vi "GoTo.vi"(6 "Reinitialize":bool, 10 "Target":dbl[](array[numeric]), 11 "Position":dbl[](array[numeric])) -> (3 "Output\nVelocity":dbl[](array[numeric]) format="%.2f")   [LabVIEW 2016]
uses:
  <vilib>/Analysis/coordinate.llb/2D Cartesian Coordinate Rotation (Scalar).vi
  <vilib>/addons/control/pid/pid.llb/PID (DBL Array).vi
  <vilib>/addons/control/pid/NI_PID_pid.lvlib
  <vilib>/Analysis/NI_AALPro.lvlib
panel:
  out "ERROR W":dbl(graph)
  out "ERROR Y":dbl(graph)
  out "ERROR X":dbl(graph)
  in  "output range":cluster{"output high":dbl, "output low":dbl}[](array[cluster])=[{"output high"=0.88, "output low"=-0.88}, {"output high"=0.88, "output low"=-0.88}, {"output high"=1.0, "output low"=-1.0}]
  in  "PID gains":T1(array[cluster])=[{"proportional gain (Kc)"=0.0012, "integral time (Ti, min)"=0.0, "derivative time (Td, min)"=0.0}, {"proportional gain (Kc)"=1.5, "integral time (Ti, min)"=0.0, "derivative time (Td, min)"=0.0}]
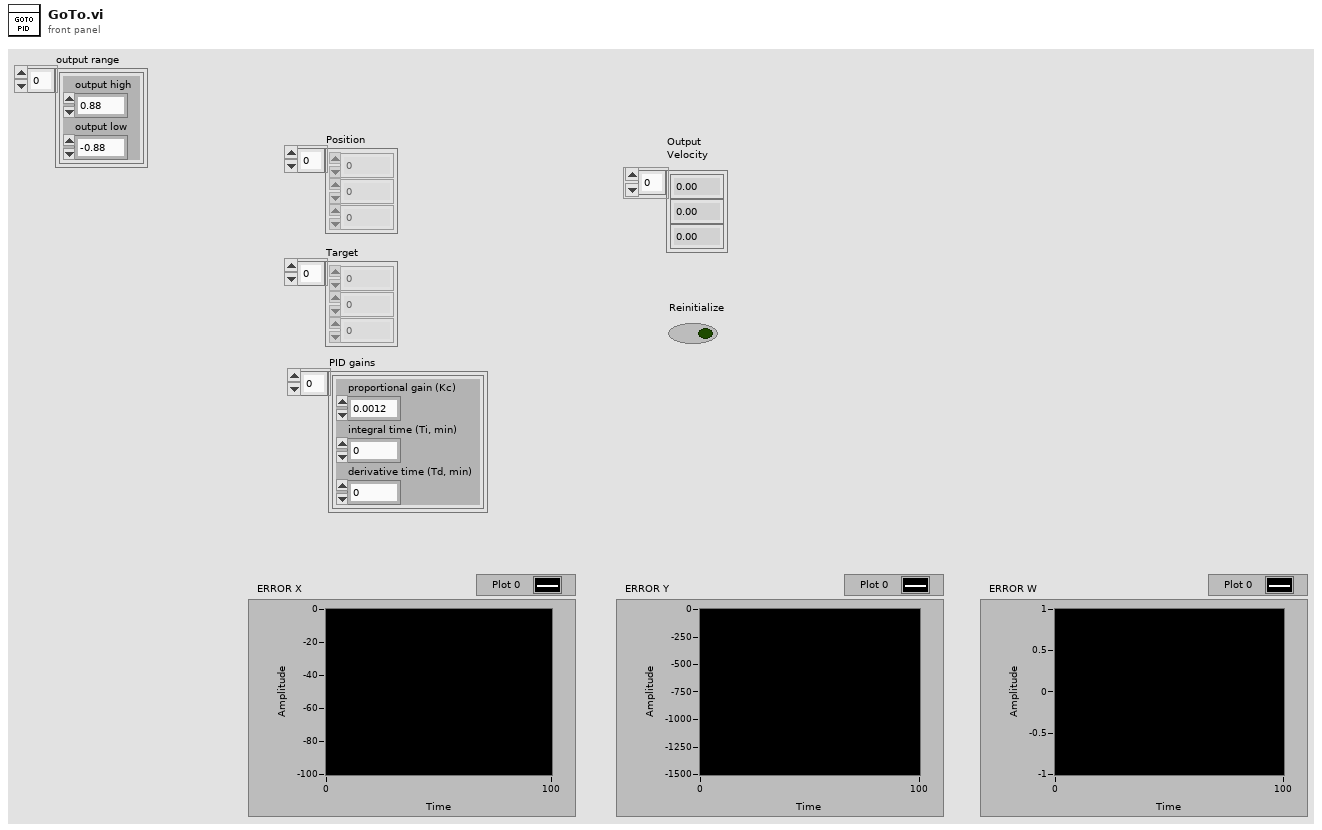
[diagram p1: front panel]
types:
  T1 = cluster{"proportional gain (Kc)":dbl, "integral time (Ti, min)":dbl, "derivative time (Td, min)":dbl}[]
  T2 = cluster{"proportional gain (Kc)":dbl, "integral time (Ti, min)":dbl, "derivative time (Td, min)":dbl}
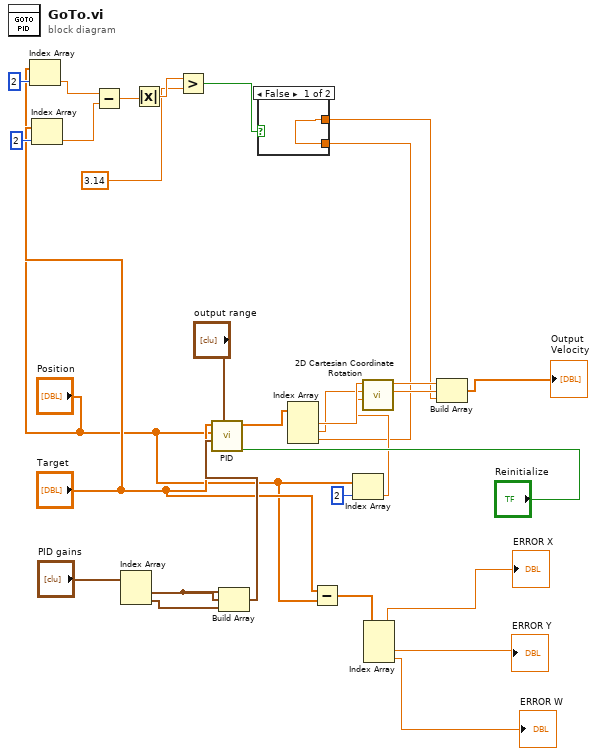
[diagram p0: block diagram]
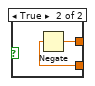
[diagram p2: hidden frame]
diagram:
  n1 = Index Array(array="Position", index=2) -> (element=w14:dbl)
  n2 = Index Array(array="Target", index=2) -> (element=w13:dbl)
  n3 = Subtract(x=w14, y=w13) -> (x-y=w12:dbl)
  n4 = Index Array(array="PID gains") -> (element #1=w19:T2, element #2=w18:T2)  [unwired: 2 in]
  n5 = Absolute Value(x=w12) -> (abs(x)=w11:dbl)
  n6 = Greater?(x=w11, y=3.14) -> (0:w9:bool)
  n7 = Build Array(w19, w19, w18) -> (w17:T1)
  n8 = call-poly <vilib>:"PID.vi"("reinitialize? (F)"="Reinitialize", "output range"="output range", "PID gains"=w17, "process variable"="Position", "setpoint"="Target") -> ("output"=w28:dbl[])  [unwired: 5 in, 1 out]
  n9 = Index Array(array=w28) -> (element #1=w27:dbl, element #2=w26:dbl, element #3=w8:dbl)  [unwired: 3 in]
  n10 = case shown="False" w9 {
    tunnel: w8 -> [w31 w33]
    tunnel: [w31 w32] -> w7
    frame False {
    }
    frame True {
      n11 = Negate(x=w33) -> (-x=w32:dbl)
    }
  }
  n12 = Subtract(x="Target", y="Position") -> (x-y=w4:dbl[])
  n13 = Index Array(array="Position", index=2) -> (element=w21:dbl)
  n14 = call-poly <vilib>:"2D Cartesian Coordinate Rotation.vi"("theta"=w21, "y"=w26, "x"=w27) -> ("y out"=w24:dbl, "x out"=w25:dbl)  [unwired: 6 in, 1 out]
  n15 = Index Array(array=w4) -> (element #1=→"ERROR X":dbl, element #2=→"ERROR Y":dbl, element #3=→"ERROR W":dbl)  [unwired: 3 in]
  n16 = Build Array(w25, w24, w7) -> (→"Output\nVelocity":dbl[])
